vi "Autonomous Independent.vi"   [LabVIEW 2016]
doc: "This VI is called when autonomous begins, and will automatically be terminated when autonomous ends. You can carry out timed or sensor driven robot movement independently without needing to return to the caller."
uses:
  <vilib>/Rock Robotics/WPI/Solenoid/WPI_SolenoidValue.ctl
  <vilib>/Rock Robotics/WPI/Utilities/WPI_GetSetVariantRefNum.vi
  <vilib>/Rock Robotics/Network Tables/NT Read String.vi
  <vilib>/Rock Robotics/Network Tables/NT Write Numeric Array.vi
  <vilib>/Rock Robotics/Network Tables/NT Read Number.vi
  <vilib>/Rock Robotics/WPI/RobotDrive/WPI_RobotDriveArcadeDrive_Standard(NoSaturation).vi
  <vilib>/Rock Robotics/Network Tables/NT Write Number.vi
  <vilib>/Rock Robotics/Network Tables/NT Write String.vi
  <vilib>/Rock Robotics/WPI/Solenoid/WPI_SolenoidSetEnum.vi
  test2/Robot Global Data.vi
panel:
  # "Be sure to right-click and choose Data Operations>>Make Current Value default if you want to save the array values with the VI"
types:
  T1 = typedef "WPI_JoystickDevRef.ctl" = cluster{"Device":T2}
  T2 = typedef "WPI_JoystickDeviceEnum.ctl" = enum16{"USB 0", "USB 1", "USB 2", "USB 3", "USB 4", "USB 5"}
  T3 = typedef "WPI_EncoderDevRef.ctl" = cluster{"DevStatus":errorcluster, "EncoderIndex":T4, "CounterIndex":T5, "DistancePerCount":dbl, "Decoding Type":T6}
  T4 = typedef "FPGA_EncoderIdx.ctl" = enum8{"Enc 0", "Enc 1", "Enc 2", "Enc 3", "Enc 4", "Enc 5", "Enc 6", "Enc 7", "Invalid"}
  T5 = typedef "FPGA_CounterCtrSystemIndex.ctl" = enum8{"Ctr 0", "Ctr 1", "Ctr 2", "Ctr 3", "Ctr 4", "Ctr 5", "Ctr 6", "Ctr 7", "Invalid"}
  T6 = typedef "WPI_EncoderType.ctl" = enum16{"1x", "2x", "4x"}
  T7 = typedef "WPI_RobotDriveDevRef.ctl" = cluster{"DevStatus":errorcluster, "Motors[]":T8[], "Square Inputs":bool, "Max Output":dbl}
  T8 = typedef "WPI_MotorControlDeviceRef.ctl" = cluster{"DeviceStatus":errorcluster, "Type":T9, "PWM":cluster{"PWM Channel":T10, "DeadBand":T11}, "CAN":cluster{"Device Number":u8, "SetOutput VI Ref":variant, "GetOutput VI Ref":variant, "Enable VI Ref":variant, "Disable VI Ref":variant, "Data":variant}, "Invert":bool}
  T9 = typedef "WPI_MotorControlType.ctl" = enum16{"PWM", "CAN"}
  T10 = typedef "FPGA_DIOPWMChannel.ctl" = enum8{"PWM 0", "PWM 1", "PWM 2", "PWM 3", "PWM 4", "PWM 5", "PWM 6", "PWM 7", "PWM 8", "PWM 9", "PWM MXP 0", "PWM MXP 1", "PWM MXP 2", "PWM MXP 3", "PWM MXP 4", "PWM MXP 5", "PWM MXP 6", "PWM MXP 7", "PWM MXP 8", "PWM MXP 9", "Invalid"}
  T11 = typedef "WPI_PWMDeadband.ctl" = cluster{"Name":string, "maxPositivePwm":i32, "minPositivePwm":i32, "centerPwm":i32, "maxNegativePwm":i32, "minNegativePwm":i32, "angularRange":u16}
  T12 = typedef "WPI_GyroDevRef.ctl" = cluster{"DevStatus":errorcluster, "Analog Channel":T13, "Offset":dbl, "Gain (VoltsPerDegree/Second)":dbl, "Gyro Type":enum16{"Analog", "XRS450"}, "Handle":i32, "SPI Bus":T14, "Device Found":bool, "Sample Rate":dbl, "Calibrate On Open":bool}
  T13 = typedef "FPGA_AIChannel.ctl" = enum8{"AI 0", "AI 1", "AI 2", "AI 3", "AI MXP 0", "AI MXP 1", "AI MXP 2", "AI MXP 3", "Invalid"}
  T14 = typedef "spi_bus.ctl" = enum16{"SPI On-Board, CS0", "SPI On-Board, CS1", "SPI On-Board, CS2", "SPI On-Board, CS3", "SPI MXP", "Invalid"}
  T15 = typedef "WPI_SolenoidValue.ctl" = enum16{"Off", "On", "Forward", "Reverse"}
  T16 = typedef "WPI_SolenoidDevRef.ctl" = cluster{"DevStatus":errorcluster, "Pneumatics Control Module":u8, "Forward Solenoid Channel":T17, "Reverse Solenoid Channel":T17}
  T17 = typedef "WPI_SolenoidChannel.ctl" = enum8{"Solenoid 0", "Solenoid 1", "Solenoid 2", "Solenoid 3", "Solenoid 4", "Solenoid 5", "Solenoid 6", "Solenoid 7", "Invalid"}
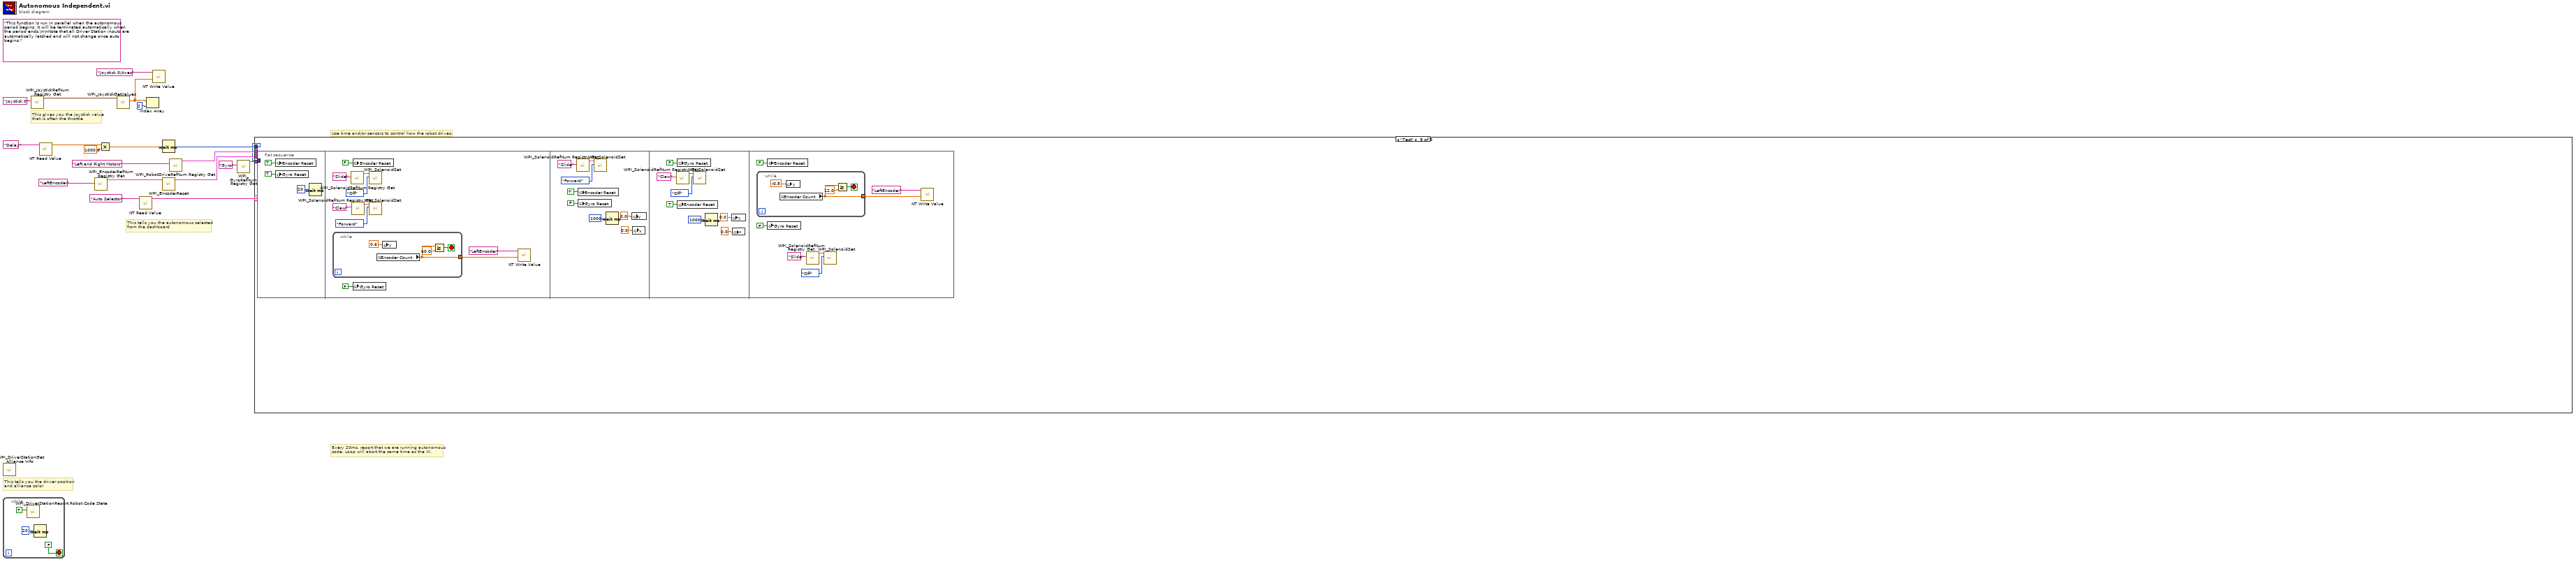
[diagram p0: block diagram]
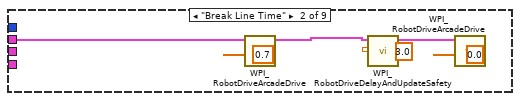
[diagram p3: hidden frame]
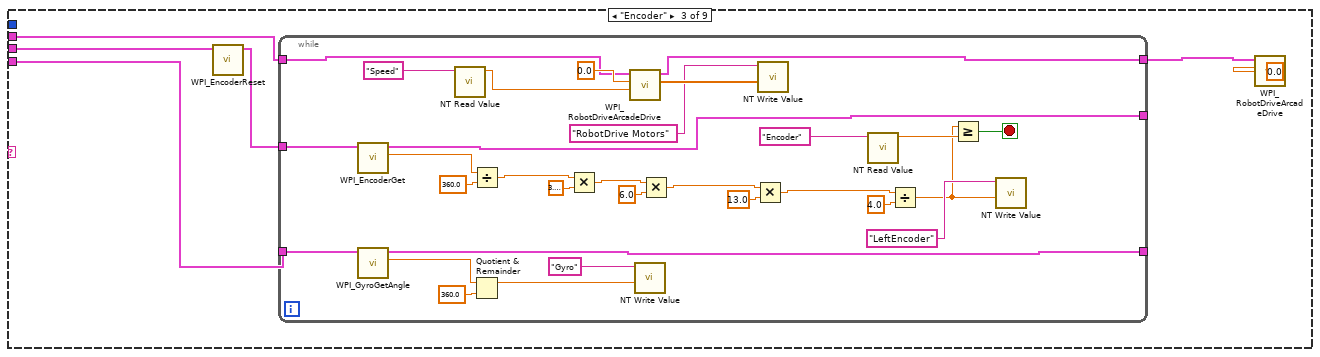
[diagram p4: hidden frame]
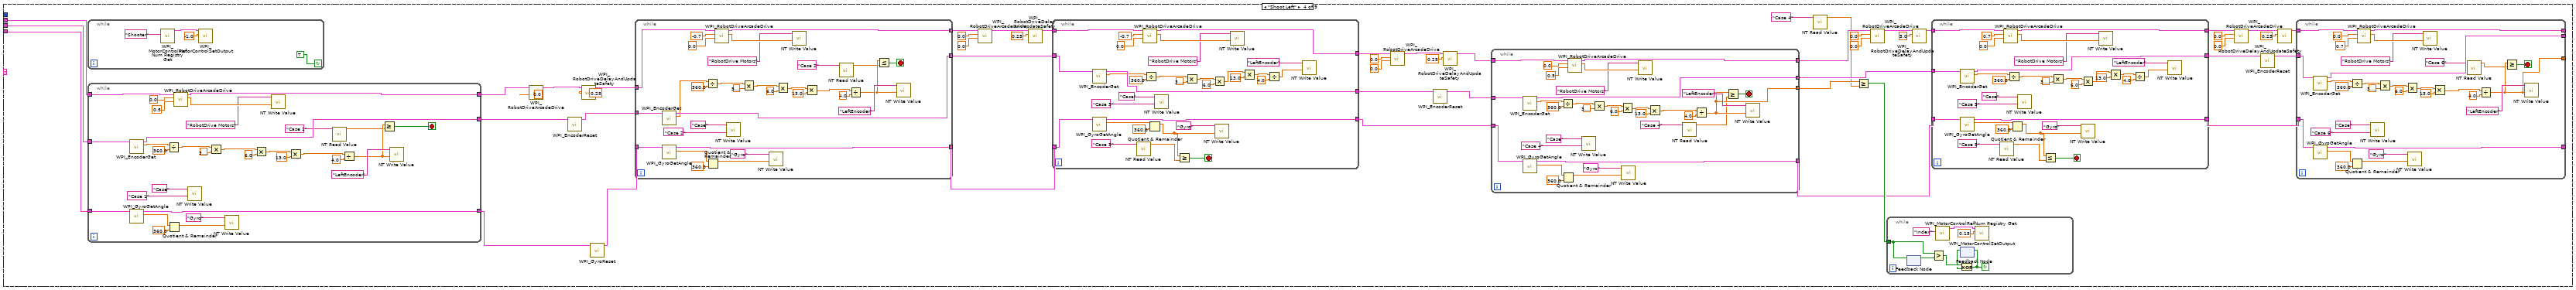
[diagram p5: hidden frame]
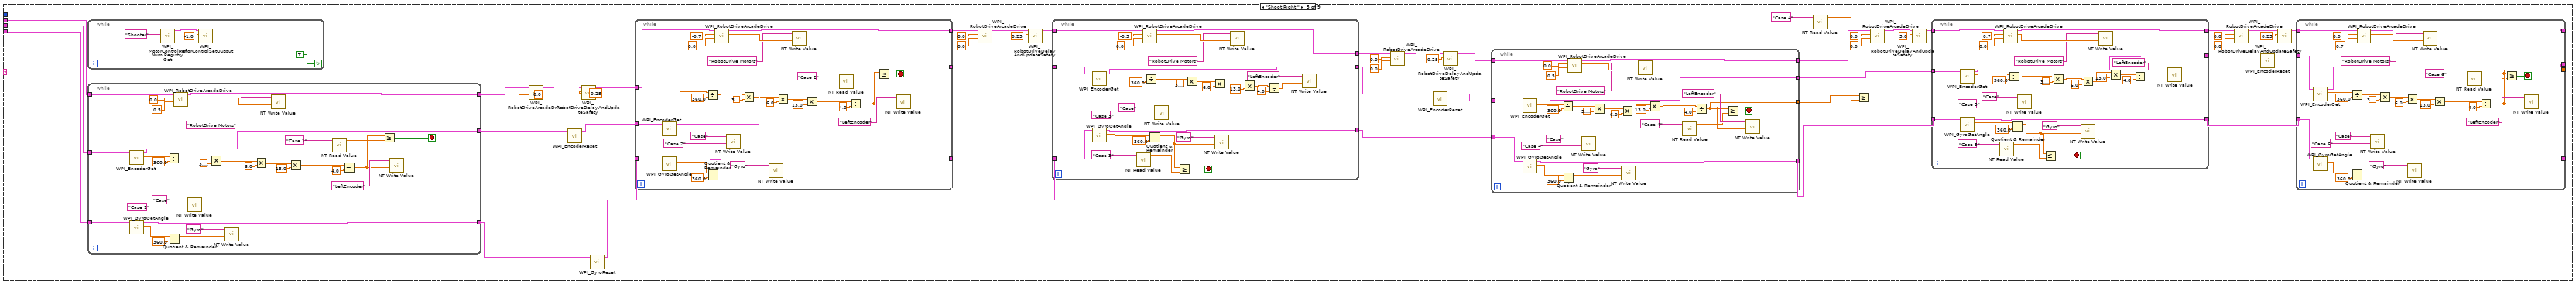
[diagram p6: hidden frame]
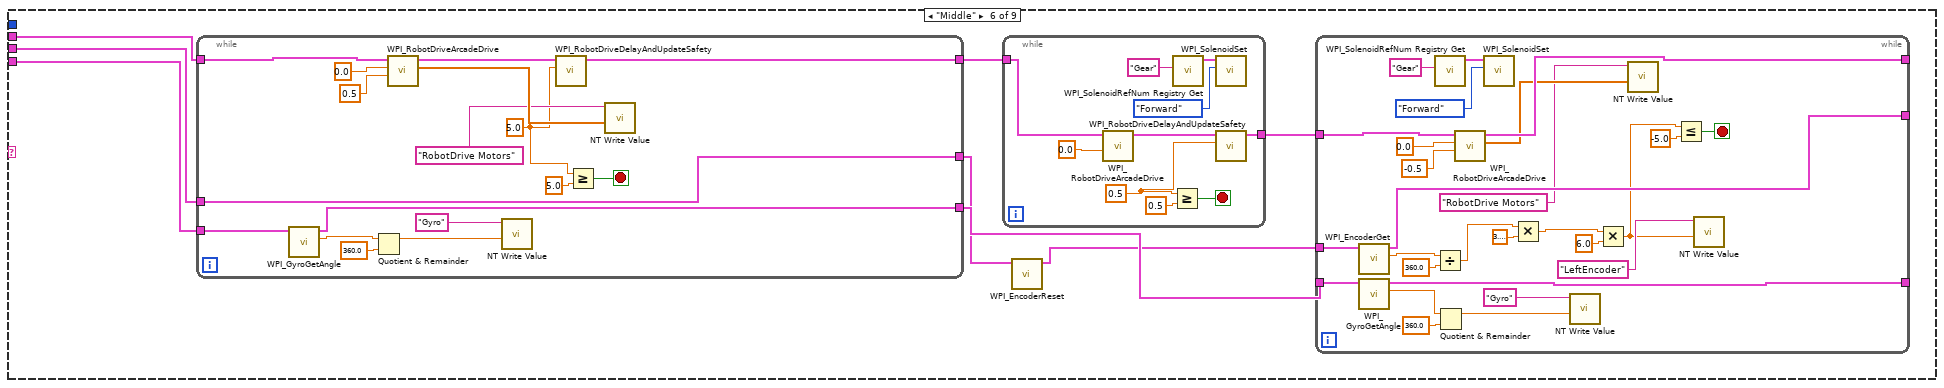
[diagram p7: hidden frame]
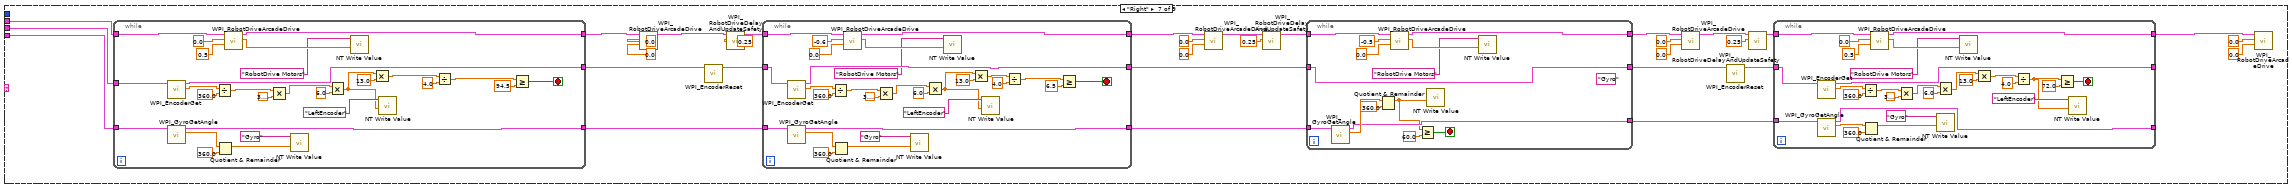
[diagram p8: hidden frame]
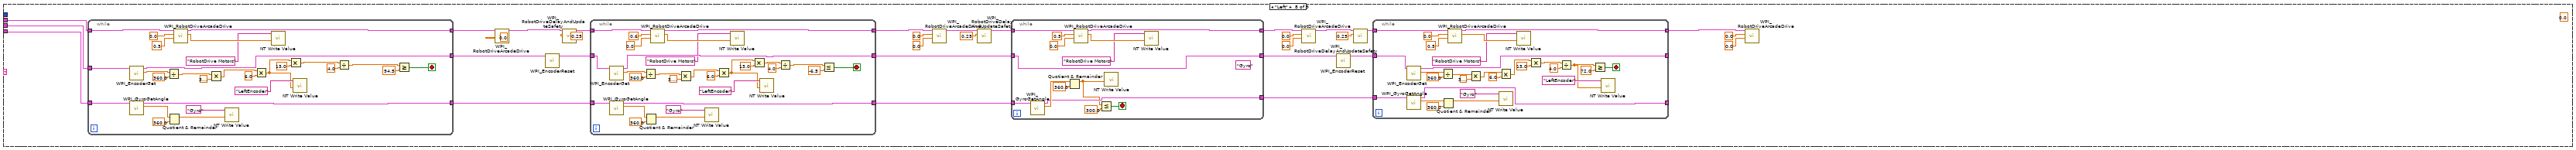
[diagram p9: hidden frame]
diagram:
  (unwired) "This function is run in parallel when the autonomous period begins. It will be terminated automatically when the period ends.\n\nNote that all Driver Station inputs are automatically latched and will not change once auto begins."
  # "This tells you the autonomous selected\nfrom the dashboard"
  # "Every 20ms, report that we are running autonomous\ncode. Loop will abort the same time as the VI."
  # "This gives you the joystick value\nthat is often the throttle"
  # "Use time and/or sensors to control how the robot drives."
  # "This tells you the driver position\nand alliance color"
  n1 = call <vilib>:"WPI_DriverStationGet Alliance Info.vi"() -> ()  [unwired: 12 out]
  n2 = while {
    stop <- FALSE stop-if-true
    n3 = call <vilib>:"WPI_DriverStationReport Robot Code State.vi"("Autonomous"=TRUE) -> ()  [unwired: 10 in, 1 out]
    n4 = Wait (ms)(milliseconds to wait=u32 20) -> ()  [unwired: 1 out]
  }
  n5 = call <vilib>:"WPI_JoystickRefNum Registry Get.vi"("refnum name"="Joystick 0") -> ("JoystickDevRef"=w18:T1)  [unwired: 1 in, 9 out]
  n6 = call-poly <vilib>:"NT Read Value.vi"("Name"="Delay") -> ("Numeric"=w7:dbl)  [unwired: 9 in, 1 out]
  n7 = call <vilib>:"WPI_EncoderRefNum Registry Get.vi"("refnum name"="LeftEncoder") -> ("EncoderDevRef"=w9:T3)  [unwired: 9 in, 1 out]
  n8 = Multiply(x=w7, y=1000.0) -> (x*y=w5:dbl)
  n9 = call <vilib>:"WPI_JoystickGetValues.vi"("JoystickDevRef"=w18) -> ("Axes"=w14:dbl[])  [unwired: 6 in, 4 out]
  n10 = call-poly <vilib>:"NT Read Value.vi"("Name"="Auto Selector") -> ("String"=w15:string)  [unwired: 9 in, 1 out]
  n11 = Index Array(array=w14, index=2) -> ()  [unwired: 1 out]
  n12 = call-poly <vilib>:"NT Write Value.vi"("Numeric Array"=w14, "Name"="Joystick 0/Axes") -> ()  [unwired: 9 in, 1 out]
  n13 = Wait (ms)(milliseconds to wait=w5) -> (millisecond timer value=w8:u32)
  n14 = call <vilib>:"WPI_EncoderReset.vi"("EncoderDevRef"=w9) -> ("EncoderDevRef"=w1:T3)  [unwired: 9 in, 1 out]
  n15 = call <vilib>:"WPI_RobotDriveRefNum Registry Get.vi"("refnum name"="Left and Right Motors") -> ("RobotDriveDevRef"=w3:T7)  [unwired: 1 in, 9 out]
  n16 = call <vilib>:"WPI_GyroRefNum Registry Get.vi"("refnum name"="Gyro") -> ("GyroDevRef"=w2:T12)  [unwired: 9 in, 1 out]
  n17 = case shown="\"Test\"" w15 {
    tunnel: w8 -> [_ _ _ _ _ _ _ _ w873]
    tunnel: w3 -> [_ w23 w33 w109 w315 w555 w626 w746 _]
    tunnel: w2 -> [_ _ w34 w108 w314 w554 w625 w745 _]
    tunnel: w1 -> [_ _ w32 w107 w313 w553 w624 w744 _]
    frame Default {
      # "You can put your main auto here, or you can right-click on the case and make any\nother frame be the default case."
      # "This is the frame that will execute if no selection is made, or if it is not recognized"
    }
    frame "Break Line Time" {
      n18 = call-poly <vilib>:"WPI_RobotDriveArcadeDrive.vi"("Y axis value"=0.7, "RobotDriveDevRef"=w23) -> ("RobotDriveDevRef"=w27:T7)  [unwired: 7 in, 2 out]
      n19 = call <vilib>:"WPI_RobotDriveDelayAndUpdateSafety.vi"("Delay (s)"=3.0, "RobotDriveDevRef"=w27) -> ("RobotDriveDevRef 2"=w25:T7)  [unwired: 8 in, 1 out]
      n20 = call-poly <vilib>:"WPI_RobotDriveArcadeDrive.vi"("Y axis value"=0.0, "RobotDriveDevRef"=w25) -> ()  [unwired: 7 in, 3 out]
    }
    frame "Encoder" {
      n21 = call <vilib>:"WPI_EncoderReset.vi"("EncoderDevRef"=w32) -> ("EncoderDevRef"=w29:T3)  [unwired: 9 in, 1 out]
      n22 = while {
        tunnel: [w62] -> _
        tunnel: [w61] -> w31
        tunnel: w33 -> [w43]
        tunnel: w34 -> [w42]
        tunnel: w29 -> [w41]
        tunnel: [w40] -> _
        stop <- w44 stop-if-true
        n23 = call <vilib>:"WPI_EncoderGet.vi"("EncoderDevRef"=w41) -> ("Distance"=w52:dbl, "EncoderDevRef"=w40:T3)  [unwired: 5 in, 4 out]
        n24 = call <vilib>:"WPI_GyroGetAngle.vi"("GyroDevRef"=w42) -> ("Angle"=w64:dbl, "GyroDevRef"=w62:T12)  [unwired: 6 in, 3 out]
        n25 = call-poly <vilib>:"NT Read Value.vi"("Name"="Speed") -> ("Numeric"=w35:dbl)  [unwired: 9 in, 1 out]
        n26 = Divide(x=w52, y=360.0) -> (x/y=w50:dbl)
        n27 = Quotient & Remainder(x=w64, y=360.0) -> (x-y*floor(x/y)=w60:dbl)  [unwired: 1 out]
        n28 = Multiply(x=w50, y=3.141592653589793) -> (x*y=w54:dbl)
        n29 = call-poly <vilib>:"WPI_RobotDriveArcadeDrive.vi"("Y axis value"=w35, "X axis value"=0.0, "RobotDriveDevRef"=w43) -> ("Motor Values"=w58:dbl[], "RobotDriveDevRef"=w61:T7)  [unwired: 6 in, 1 out]
        n30 = call-poly <vilib>:"NT Write Value.vi"("Numeric"=w60, "Name"="Gyro") -> ()  [unwired: 9 in, 1 out]
        n31 = Multiply(x=w54, y=6.0) -> (x*y=w45:dbl)
        n32 = Multiply(x=w45, y=13.0) -> (x*y=w46:dbl)
        n33 = call-poly <vilib>:"NT Write Value.vi"("Numeric Array"=w58, "Name"="RobotDrive Motors") -> ()  [unwired: 9 in, 1 out]
        n34 = call-poly <vilib>:"NT Read Value.vi"("Name"="Encoder") -> ("Numeric"=w39:dbl)  [unwired: 9 in, 1 out]
        n35 = Divide(x=w46, y=4.0) -> (x/y=w37:dbl)
        n36 = Greater Or Equal?(x=w37, y=w39) -> (x >= y?=w44:bool)
        n37 = call-poly <vilib>:"NT Write Value.vi"("Numeric"=w37, "Name"="LeftEncoder") -> ()  [unwired: 9 in, 1 out]
      }
      n38 = call-poly <vilib>:"WPI_RobotDriveArcadeDrive.vi"("X axis value"=0.0, "RobotDriveDevRef"=w31) -> ()  [unwired: 7 in, 3 out]
    }
    frame "Shoot Left" {
      n39 = while {
        stop <- TRUE ("x") continue-if-true
        n40 = call <vilib>:"WPI_MotorControlRefNum Registry Get.vi"("refnum name"="Shooter") -> ("MotorControlDevRef"=w179:T8)  [unwired: 9 in, 1 out]
        n41 = call <vilib>:"WPI_MotorControlSetOutput.vi"("Output"=-1.0, "MotorControlDevRef"=w179) -> ()  [unwired: 7 in, 3 out]
      }
      n42 = while {
        tunnel: [w308] -> w114
        tunnel: [w307] -> w96
        tunnel: [w306] -> w112
        tunnel: w109 -> [w289]
        tunnel: w108 -> [w288]
        tunnel: w107 -> [w287]
        stop <- w309 stop-if-true
        n43 = call <vilib>:"WPI_EncoderGet.vi"("EncoderDevRef"=w287) -> ("Distance"=w297:dbl, "EncoderDevRef"=w308:T3)  [unwired: 5 in, 4 out]
        n44 = call <vilib>:"WPI_GyroGetAngle.vi"("GyroDevRef"=w288) -> ("Angle"=w311:dbl, "GyroDevRef"=w307:T12)  [unwired: 6 in, 3 out]
        n45 = Divide(x=w297, y=360.0) -> (x/y=w295:dbl)
        n46 = Quotient & Remainder(x=w311, y=360.0) -> (x-y*floor(x/y)=w305:dbl)  [unwired: 1 out]
        n47 = call-poly <vilib>:"WPI_RobotDriveArcadeDrive.vi"("Y axis value"=0.5, "X axis value"=0.0, "RobotDriveDevRef"=w289) -> ("Motor Values"=w303:dbl[], "RobotDriveDevRef"=w306:T7)  [unwired: 6 in, 1 out]
        n48 = call-poly <vilib>:"NT Write Value.vi"("String"="Case 1", "Name"="Case") -> ()  [unwired: 9 in, 1 out]
        n49 = Multiply(x=w295, y=3.141592653589793) -> (x*y=w299:dbl)
        n50 = call-poly <vilib>:"NT Write Value.vi"("Numeric"=w305, "Name"="Gyro") -> ()  [unwired: 9 in, 1 out]
        n51 = Multiply(x=w299, y=6.0) -> (x*y=w290:dbl)
        n52 = call-poly <vilib>:"NT Write Value.vi"("Numeric Array"=w303, "Name"="RobotDrive Motors") -> ()  [unwired: 9 in, 1 out]
        n53 = Multiply(x=w290, y=13.0) -> (x*y=w291:dbl)
        n54 = call-poly <vilib>:"NT Read Value.vi"("Name"="Case 1") -> ("Numeric"=w284:dbl)  [unwired: 9 in, 1 out]
        n55 = Divide(x=w291, y=4.0) -> (x/y=w286:dbl)
        n56 = Greater Or Equal?(x=w286, y=w284) -> (x >= y?=w309:bool)
        n57 = call-poly <vilib>:"NT Write Value.vi"("Numeric"=w286, "Name"="LeftEncoder") -> ()  [unwired: 9 in, 1 out]
      }
      n58 = call-poly <vilib>:"WPI_RobotDriveArcadeDrive.vi"("Y axis value"=0.0, "RobotDriveDevRef"=w112) -> ("RobotDriveDevRef"=w111:T7)  [unwired: 7 in, 2 out]
      n59 = call <vilib>:"WPI_EncoderReset.vi"("EncoderDevRef"=w114) -> ("EncoderDevRef"=w105:T3)  [unwired: 9 in, 1 out]
      n60 = call <vilib>:"WPI_RobotDriveDelayAndUpdateSafety.vi"("Delay (s)"=0.25, "RobotDriveDevRef"=w111) -> ("RobotDriveDevRef 2"=w106:T7)  [unwired: 8 in, 1 out]
      n61 = call <vilib>:"WPI_GyroReset.vi"("GyroDevRef"=w96) -> ("GyroDevRef"=w95:T12)  [unwired: 9 in, 1 out]
      n62 = while {
        tunnel: [w278] -> w97
        tunnel: [w277] -> w98
        tunnel: [w276] -> w101
        tunnel: w106 -> [w259]
        tunnel: w95 -> [w258]
        tunnel: w105 -> [w257]
        stop <- w255 stop-if-true
        n63 = call <vilib>:"WPI_EncoderGet.vi"("EncoderDevRef"=w257) -> ("Distance"=w267:dbl, "EncoderDevRef"=w278:T3)  [unwired: 5 in, 4 out]
        n64 = call <vilib>:"WPI_GyroGetAngle.vi"("GyroDevRef"=w258) -> ("Angle"=w280:dbl, "GyroDevRef"=w277:T12)  [unwired: 6 in, 3 out]
        n65 = Divide(x=w267, y=360.0) -> (x/y=w265:dbl)
        n66 = Quotient & Remainder(x=w280, y=360.0) -> (x-y*floor(x/y)=w275:dbl)  [unwired: 1 out]
        n67 = call-poly <vilib>:"WPI_RobotDriveArcadeDrive.vi"("Y axis value"=0.0, "X axis value"=-0.7, "RobotDriveDevRef"=w259) -> ("Motor Values"=w273:dbl[], "RobotDriveDevRef"=w276:T7)  [unwired: 6 in, 1 out]
        n68 = call-poly <vilib>:"NT Write Value.vi"("String"="Case 2", "Name"="Case") -> ()  [unwired: 9 in, 1 out]
        n69 = Multiply(x=w265, y=3.141592653589793) -> (x*y=w269:dbl)
        n70 = call-poly <vilib>:"NT Write Value.vi"("Numeric"=w275, "Name"="Gyro") -> ()  [unwired: 9 in, 1 out]
        n71 = Multiply(x=w269, y=6.0) -> (x*y=w260:dbl)
        n72 = call-poly <vilib>:"NT Write Value.vi"("Numeric Array"=w273, "Name"="RobotDrive Motors") -> ()  [unwired: 9 in, 1 out]
        n73 = Multiply(x=w260, y=13.0) -> (x*y=w261:dbl)
        n74 = call-poly <vilib>:"NT Read Value.vi"("Name"="Case 2") -> ("Numeric"=w253:dbl)  [unwired: 9 in, 1 out]
        n75 = Divide(x=w261, y=4.0) -> (x/y=w256:dbl)
        n76 = Less Or Equal?(x=w256, y=w253) -> (x <= y?=w255:bool)
        n77 = call-poly <vilib>:"NT Write Value.vi"("Numeric"=w256, "Name"="LeftEncoder") -> ()  [unwired: 9 in, 1 out]
      }
      n78 = call-poly <vilib>:"WPI_RobotDriveArcadeDrive.vi"("Y axis value"=0.0, "X axis value"=0.0, "RobotDriveDevRef"=w101) -> ("RobotDriveDevRef"=w103:T7)  [unwired: 6 in, 2 out]
      n79 = call <vilib>:"WPI_RobotDriveDelayAndUpdateSafety.vi"("Delay (s)"=0.25, "RobotDriveDevRef"=w103) -> ("RobotDriveDevRef 2"=w99:T7)  [unwired: 8 in, 1 out]
      n80 = while {
        tunnel: [w246] -> w87
        tunnel: [w245] -> w88
        tunnel: [w244] -> w89
        tunnel: w99 -> [w228]
        tunnel: w98 -> [w227]
        tunnel: w97 -> [w226]
        stop <- w247 stop-if-true
        n81 = call <vilib>:"WPI_EncoderGet.vi"("EncoderDevRef"=w226) -> ("Distance"=w236:dbl, "EncoderDevRef"=w246:T3)  [unwired: 5 in, 4 out]
        n82 = call <vilib>:"WPI_GyroGetAngle.vi"("GyroDevRef"=w227) -> ("Angle"=w249:dbl, "GyroDevRef"=w245:T12)  [unwired: 6 in, 3 out]
        n83 = call-poly <vilib>:"NT Read Value.vi"("Name"="Case 3") -> ("Numeric"=w222:dbl)  [unwired: 9 in, 1 out]
        n84 = call-poly <vilib>:"WPI_RobotDriveArcadeDrive.vi"("Y axis value"=0.0, "X axis value"=-0.7, "RobotDriveDevRef"=w228) -> ("Motor Values"=w242:dbl[], "RobotDriveDevRef"=w244:T7)  [unwired: 6 in, 1 out]
        n85 = Divide(x=w236, y=360.0) -> (x/y=w234:dbl)
        n86 = Quotient & Remainder(x=w249, y=360.0) -> (x-y*floor(x/y)=w224:dbl)  [unwired: 1 out]
        n87 = call-poly <vilib>:"NT Write Value.vi"("String"="Case 3", "Name"="Case") -> ()  [unwired: 9 in, 1 out]
        n88 = Greater Or Equal?(x=w224, y=w222) -> (x >= y?=w247:bool)
        n89 = Multiply(x=w234, y=3.141592653589793) -> (x*y=w238:dbl)
        n90 = Multiply(x=w238, y=6.0) -> (x*y=w229:dbl)
        n91 = call-poly <vilib>:"NT Write Value.vi"("Numeric"=w224, "Name"="Gyro") -> ()  [unwired: 9 in, 1 out]
        n92 = call-poly <vilib>:"NT Write Value.vi"("Numeric Array"=w242, "Name"="RobotDrive Motors") -> ()  [unwired: 9 in, 1 out]
        n93 = Multiply(x=w229, y=13.0) -> (x*y=w230:dbl)
        n94 = Divide(x=w230, y=4.0) -> (x/y=w225:dbl)
        n95 = call-poly <vilib>:"NT Write Value.vi"("Numeric"=w225, "Name"="LeftEncoder") -> ()  [unwired: 9 in, 1 out]
      }
      n96 = call-poly <vilib>:"WPI_RobotDriveArcadeDrive.vi"("Y axis value"=0.0, "X axis value"=0.0, "RobotDriveDevRef"=w89) -> ("RobotDriveDevRef"=w93:T7)  [unwired: 6 in, 2 out]
      n97 = call <vilib>:"WPI_EncoderReset.vi"("EncoderDevRef"=w87) -> ("EncoderDevRef"=w86:T3)  [unwired: 9 in, 1 out]
      n98 = call <vilib>:"WPI_RobotDriveDelayAndUpdateSafety.vi"("Delay (s)"=0.25, "RobotDriveDevRef"=w93) -> ("RobotDriveDevRef 2"=w90:T7)  [unwired: 8 in, 1 out]
      n99 = while {
        tunnel: [w216] -> w82
        tunnel: [w215] -> w83
        tunnel: [w214] -> w78
        tunnel: w90 -> [w197]
        tunnel: w88 -> [w196]
        tunnel: w86 -> [w195]
        tunnel: [w193] -> w85
        stop <- w194 stop-if-true
        n100 = call <vilib>:"WPI_EncoderGet.vi"("EncoderDevRef"=w195) -> ("Distance"=w205:dbl, "EncoderDevRef"=w216:T3)  [unwired: 5 in, 4 out]
        n101 = call <vilib>:"WPI_GyroGetAngle.vi"("GyroDevRef"=w196) -> ("Angle"=w218:dbl, "GyroDevRef"=w215:T12)  [unwired: 6 in, 3 out]
        n102 = Divide(x=w205, y=360.0) -> (x/y=w203:dbl)
        n103 = Quotient & Remainder(x=w218, y=360.0) -> (x-y*floor(x/y)=w213:dbl)  [unwired: 1 out]
        n104 = call-poly <vilib>:"WPI_RobotDriveArcadeDrive.vi"("Y axis value"=0.5, "X axis value"=0.0, "RobotDriveDevRef"=w197) -> ("Motor Values"=w211:dbl[], "RobotDriveDevRef"=w214:T7)  [unwired: 6 in, 1 out]
        n105 = call-poly <vilib>:"NT Write Value.vi"("String"="Case 4", "Name"="Case") -> ()  [unwired: 9 in, 1 out]
        n106 = Multiply(x=w203, y=3.141592653589793) -> (x*y=w207:dbl)
        n107 = Multiply(x=w207, y=6.0) -> (x*y=w198:dbl)
        n108 = call-poly <vilib>:"NT Write Value.vi"("Numeric"=w213, "Name"="Gyro") -> ()  [unwired: 9 in, 1 out]
        n109 = call-poly <vilib>:"NT Write Value.vi"("Numeric Array"=w211, "Name"="RobotDrive Motors") -> ()  [unwired: 9 in, 1 out]
        n110 = Multiply(x=w198, y=13.0) -> (x*y=w199:dbl)
        n111 = call-poly <vilib>:"NT Read Value.vi"("Name"="Case 4") -> ("Numeric"=w191:dbl)  [unwired: 9 in, 1 out]
        n112 = Divide(x=w199, y=4.0) -> (x/y=w193:dbl)
        n113 = Greater Or Equal?(x=w193, y=w191) -> (x >= y?=w194:bool)
        n114 = call-poly <vilib>:"NT Write Value.vi"("Numeric"=w193, "Name"="LeftEncoder") -> ()  [unwired: 9 in, 1 out]
      }
      n115 = call-poly <vilib>:"NT Read Value.vi"("Name"="Case 4") -> ("Numeric"=w65:dbl)  [unwired: 9 in, 1 out]
      n116 = Greater Or Equal?(x=w85, y=w65) -> (x >= y?=w84:bool)
      n117 = call-poly <vilib>:"WPI_RobotDriveArcadeDrive.vi"("Y axis value"=0.0, "X axis value"=0.0, "RobotDriveDevRef"=w78) -> ("RobotDriveDevRef"=w80:T7)  [unwired: 6 in, 2 out]
      n118 = while {
        tunnel: w84 -> [w183]
        stop <- w182 continue-if-true
        n119 = feedback #1() -> (w186:bool)  [unwired: 1 in]
        n120 = feedback-in #1(w183) -> ()
        n121 = Greater?(x=w183, y=w186) -> (0:w185:bool)
        n122 = call <vilib>:"WPI_MotorControlRefNum Registry Get.vi"("refnum name"="Index") -> ("MotorControlDevRef"=w188:T8)  [unwired: 9 in, 1 out]
        n123 = feedback #2() -> (w184:bool)  [unwired: 1 in]
        n124 = Exclusive Or(1:w184, 2:w185) -> (0:w182:bool)
        n125 = feedback-in #2(w182) -> ()
        n126 = call <vilib>:"WPI_MotorControlSetOutput.vi"("Output"=0.15, "MotorControlDevRef"=w188) -> ()  [unwired: 7 in, 3 out]
      }
      n127 = call <vilib>:"WPI_RobotDriveDelayAndUpdateSafety.vi"("Delay (s)"=5.0, "RobotDriveDevRef"=w80) -> ("RobotDriveDevRef 2"=w76:T7)  [unwired: 8 in, 1 out]
      n128 = while {
        tunnel: [w173] -> w67
        tunnel: [w172] -> w68
        tunnel: [w171] -> w69
        tunnel: w76 -> [w155]
        tunnel: w83 -> [w154]
        tunnel: w82 -> [w151]
        stop <- w150 stop-if-true
        n129 = call <vilib>:"WPI_EncoderGet.vi"("EncoderDevRef"=w151) -> ("Distance"=w163:dbl, "EncoderDevRef"=w173:T3)  [unwired: 5 in, 4 out]
        n130 = call <vilib>:"WPI_GyroGetAngle.vi"("GyroDevRef"=w154) -> ("Angle"=w175:dbl, "GyroDevRef"=w172:T12)  [unwired: 6 in, 3 out]
        n131 = call-poly <vilib>:"NT Read Value.vi"("Name"="Case 5") -> ("Numeric"=w148:dbl)  [unwired: 9 in, 1 out]
        n132 = call-poly <vilib>:"WPI_RobotDriveArcadeDrive.vi"("Y axis value"=0.0, "X axis value"=0.7, "RobotDriveDevRef"=w155) -> ("Motor Values"=w169:dbl[], "RobotDriveDevRef"=w171:T7)  [unwired: 6 in, 1 out]
        n133 = Divide(x=w163, y=360.0) -> (x/y=w161:dbl)
        n134 = Quotient & Remainder(x=w175, y=360.0) -> (x-y*floor(x/y)=w152:dbl)  [unwired: 1 out]
        n135 = call-poly <vilib>:"NT Write Value.vi"("String"="Case 5", "Name"="Case") -> ()  [unwired: 9 in, 1 out]
        n136 = Less Or Equal?(x=w152, y=w148) -> (x <= y?=w150:bool)
        n137 = Multiply(x=w161, y=3.141592653589793) -> (x*y=w165:dbl)
        n138 = call-poly <vilib>:"NT Write Value.vi"("Numeric"=w152, "Name"="Gyro") -> ()  [unwired: 9 in, 1 out]
        n139 = Multiply(x=w165, y=6.0) -> (x*y=w156:dbl)
        n140 = call-poly <vilib>:"NT Write Value.vi"("Numeric Array"=w169, "Name"="RobotDrive Motors") -> ()  [unwired: 9 in, 1 out]
        n141 = Multiply(x=w156, y=13.0) -> (x*y=w157:dbl)
        n142 = Divide(x=w157, y=4.0) -> (x/y=w153:dbl)
        n143 = call-poly <vilib>:"NT Write Value.vi"("Numeric"=w153, "Name"="LeftEncoder") -> ()  [unwired: 9 in, 1 out]
      }
      n144 = call-poly <vilib>:"WPI_RobotDriveArcadeDrive.vi"("Y axis value"=0.0, "X axis value"=0.0, "RobotDriveDevRef"=w69) -> ("RobotDriveDevRef"=w74:T7)  [unwired: 6 in, 2 out]
      n145 = call <vilib>:"WPI_EncoderReset.vi"("EncoderDevRef"=w67) -> ("EncoderDevRef"=w70:T3)  [unwired: 9 in, 1 out]
      n146 = call <vilib>:"WPI_RobotDriveDelayAndUpdateSafety.vi"("Delay (s)"=0.25, "RobotDriveDevRef"=w74) -> ("RobotDriveDevRef 2"=w71:T7)  [unwired: 8 in, 1 out]
      n147 = while {
        tunnel: [w142] -> _
        tunnel: [w141] -> _
        tunnel: [w140] -> _
        tunnel: w71 -> [w123]
        tunnel: w68 -> [w122]
        tunnel: w70 -> [w121]
        tunnel: [w119] -> _
        stop <- w120 stop-if-true
        n148 = call <vilib>:"WPI_EncoderGet.vi"("EncoderDevRef"=w121) -> ("Distance"=w131:dbl, "EncoderDevRef"=w142:T3)  [unwired: 5 in, 4 out]
        n149 = call <vilib>:"WPI_GyroGetAngle.vi"("GyroDevRef"=w122) -> ("Angle"=w144:dbl, "GyroDevRef"=w141:T12)  [unwired: 6 in, 3 out]
        n150 = Divide(x=w131, y=360.0) -> (x/y=w129:dbl)
        n151 = Quotient & Remainder(x=w144, y=360.0) -> (x-y*floor(x/y)=w139:dbl)  [unwired: 1 out]
        n152 = call-poly <vilib>:"WPI_RobotDriveArcadeDrive.vi"("Y axis value"=0.7, "X axis value"=0.0, "RobotDriveDevRef"=w123) -> ("Motor Values"=w137:dbl[], "RobotDriveDevRef"=w140:T7)  [unwired: 6 in, 1 out]
        n153 = call-poly <vilib>:"NT Write Value.vi"("String"="Case 6", "Name"="Case") -> ()  [unwired: 9 in, 1 out]
        n154 = Multiply(x=w129, y=3.141592653589793) -> (x*y=w133:dbl)
        n155 = Multiply(x=w133, y=6.0) -> (x*y=w124:dbl)
        n156 = call-poly <vilib>:"NT Write Value.vi"("Numeric"=w139, "Name"="Gyro") -> ()  [unwired: 9 in, 1 out]
        n157 = call-poly <vilib>:"NT Write Value.vi"("Numeric Array"=w137, "Name"="RobotDrive Motors") -> ()  [unwired: 9 in, 1 out]
        n158 = Multiply(x=w124, y=13.0) -> (x*y=w125:dbl)
        n159 = call-poly <vilib>:"NT Read Value.vi"("Name"="Case 6") -> ("Numeric"=w117:dbl)  [unwired: 9 in, 1 out]
        n160 = Divide(x=w125, y=4.0) -> (x/y=w119:dbl)
        n161 = Greater Or Equal?(x=w119, y=w117) -> (x >= y?=w120:bool)
        n162 = call-poly <vilib>:"NT Write Value.vi"("Numeric"=w119, "Name"="LeftEncoder") -> ()  [unwired: 9 in, 1 out]
      }
    }
    frame "Shoot Right " {
      n163 = while {
        stop <- TRUE ("x") continue-if-true
        n164 = call <vilib>:"WPI_MotorControlRefNum Registry Get.vi"("refnum name"="Shooter") -> ("MotorControlDevRef"=w364:T8)  [unwired: 9 in, 1 out]
        n165 = call <vilib>:"WPI_MotorControlSetOutput.vi"("Output"=-1.0, "MotorControlDevRef"=w364) -> ()  [unwired: 7 in, 3 out]
      }
      n166 = while {
        tunnel: [w547] -> w361
        tunnel: [w546] -> w346
        tunnel: [w545] -> w359
        tunnel: w315 -> [w528]
        tunnel: w314 -> [w527]
        tunnel: w313 -> [w526]
        stop <- w548 stop-if-true
        n167 = call <vilib>:"WPI_EncoderGet.vi"("EncoderDevRef"=w526) -> ("Distance"=w536:dbl, "EncoderDevRef"=w547:T3)  [unwired: 5 in, 4 out]
        n168 = call <vilib>:"WPI_GyroGetAngle.vi"("GyroDevRef"=w527) -> ("Angle"=w550:dbl, "GyroDevRef"=w546:T12)  [unwired: 6 in, 3 out]
        n169 = Divide(x=w536, y=360.0) -> (x/y=w534:dbl)
        n170 = Quotient & Remainder(x=w550, y=360.0) -> (x-y*floor(x/y)=w544:dbl)  [unwired: 1 out]
        n171 = call-poly <vilib>:"WPI_RobotDriveArcadeDrive.vi"("Y axis value"=0.5, "X axis value"=0.0, "RobotDriveDevRef"=w528) -> ("Motor Values"=w542:dbl[], "RobotDriveDevRef"=w545:T7)  [unwired: 6 in, 1 out]
        n172 = call-poly <vilib>:"NT Write Value.vi"("String"="Case 1", "Name"="Case") -> ()  [unwired: 9 in, 1 out]
        n173 = Multiply(x=w534, y=3.141592653589793) -> (x*y=w538:dbl)
        n174 = call-poly <vilib>:"NT Write Value.vi"("Numeric"=w544, "Name"="Gyro") -> ()  [unwired: 9 in, 1 out]
        n175 = Multiply(x=w538, y=6.0) -> (x*y=w529:dbl)
        n176 = call-poly <vilib>:"NT Write Value.vi"("Numeric Array"=w542, "Name"="RobotDrive Motors") -> ()  [unwired: 9 in, 1 out]
        n177 = Multiply(x=w529, y=13.0) -> (x*y=w530:dbl)
        n178 = call-poly <vilib>:"NT Read Value.vi"("Name"="Case 1") -> ("Numeric"=w523:dbl)  [unwired: 9 in, 1 out]
        n179 = Divide(x=w530, y=4.0) -> (x/y=w525:dbl)
        n180 = Greater Or Equal?(x=w525, y=w523) -> (x >= y?=w548:bool)
        n181 = call-poly <vilib>:"NT Write Value.vi"("Numeric"=w525, "Name"="LeftEncoder") -> ()  [unwired: 9 in, 1 out]
      }
      n182 = call-poly <vilib>:"WPI_RobotDriveArcadeDrive.vi"("Y axis value"=0.0, "RobotDriveDevRef"=w359) -> ("RobotDriveDevRef"=w358:T7)  [unwired: 7 in, 2 out]
      n183 = call <vilib>:"WPI_EncoderReset.vi"("EncoderDevRef"=w361) -> ("EncoderDevRef"=w355:T3)  [unwired: 9 in, 1 out]
      n184 = call <vilib>:"WPI_RobotDriveDelayAndUpdateSafety.vi"("Delay (s)"=0.25, "RobotDriveDevRef"=w358) -> ("RobotDriveDevRef 2"=w356:T7)  [unwired: 8 in, 1 out]
      n185 = call <vilib>:"WPI_GyroReset.vi"("GyroDevRef"=w346) -> ("GyroDevRef"=w345:T12)  [unwired: 9 in, 1 out]
      n186 = while {
        tunnel: [w517] -> w347
        tunnel: [w516] -> w348
        tunnel: [w515] -> w351
        tunnel: w356 -> [w498]
        tunnel: w345 -> [w497]
        tunnel: w355 -> [w496]
        stop <- w494 stop-if-true
        n187 = call <vilib>:"WPI_EncoderGet.vi"("EncoderDevRef"=w496) -> ("Distance"=w506:dbl, "EncoderDevRef"=w517:T3)  [unwired: 5 in, 4 out]
        n188 = call <vilib>:"WPI_GyroGetAngle.vi"("GyroDevRef"=w497) -> ("Angle"=w519:dbl, "GyroDevRef"=w516:T12)  [unwired: 6 in, 3 out]
        n189 = Divide(x=w506, y=360.0) -> (x/y=w504:dbl)
        n190 = Quotient & Remainder(x=w519, y=360.0) -> (x-y*floor(x/y)=w514:dbl)  [unwired: 1 out]
        n191 = call-poly <vilib>:"WPI_RobotDriveArcadeDrive.vi"("Y axis value"=0.0, "X axis value"=-0.7, "RobotDriveDevRef"=w498) -> ("Motor Values"=w512:dbl[], "RobotDriveDevRef"=w515:T7)  [unwired: 6 in, 1 out]
        n192 = call-poly <vilib>:"NT Write Value.vi"("String"="Case 2", "Name"="Case") -> ()  [unwired: 9 in, 1 out]
        n193 = Multiply(x=w504, y=3.141592653589793) -> (x*y=w508:dbl)
        n194 = call-poly <vilib>:"NT Write Value.vi"("Numeric"=w514, "Name"="Gyro") -> ()  [unwired: 9 in, 1 out]
        n195 = Multiply(x=w508, y=6.0) -> (x*y=w499:dbl)
        n196 = call-poly <vilib>:"NT Write Value.vi"("Numeric Array"=w512, "Name"="RobotDrive Motors") -> ()  [unwired: 9 in, 1 out]
        n197 = Multiply(x=w499, y=13.0) -> (x*y=w500:dbl)
        n198 = call-poly <vilib>:"NT Read Value.vi"("Name"="Case 2") -> ("Numeric"=w492:dbl)  [unwired: 9 in, 1 out]
        n199 = Divide(x=w500, y=4.0) -> (x/y=w495:dbl)
        n200 = Less Or Equal?(x=w495, y=w492) -> (x <= y?=w494:bool)
        n201 = call-poly <vilib>:"NT Write Value.vi"("Numeric"=w495, "Name"="LeftEncoder") -> ()  [unwired: 9 in, 1 out]
      }
      n202 = call-poly <vilib>:"WPI_RobotDriveArcadeDrive.vi"("Y axis value"=0.0, "X axis value"=0.0, "RobotDriveDevRef"=w351) -> ("RobotDriveDevRef"=w353:T7)  [unwired: 6 in, 2 out]
      n203 = call <vilib>:"WPI_RobotDriveDelayAndUpdateSafety.vi"("Delay (s)"=0.25, "RobotDriveDevRef"=w353) -> ("RobotDriveDevRef 2"=w349:T7)  [unwired: 8 in, 1 out]
      n204 = while {
        tunnel: [w485] -> w337
        tunnel: [w484] -> w338
        tunnel: [w483] -> w339
        tunnel: w349 -> [w468]
        tunnel: w348 -> [w467]
        tunnel: w347 -> [w466]
        stop <- w486 stop-if-true
        n205 = call <vilib>:"WPI_EncoderGet.vi"("EncoderDevRef"=w466) -> ("Distance"=w459:dbl, "EncoderDevRef"=w485:T3)  [unwired: 5 in, 4 out]
        n206 = call <vilib>:"WPI_GyroGetAngle.vi"("GyroDevRef"=w467) -> ("Angle"=w488:dbl, "GyroDevRef"=w484:T12)  [unwired: 6 in, 3 out]
        n207 = call-poly <vilib>:"NT Read Value.vi"("Name"="Case 3") -> ("Numeric"=w462:dbl)  [unwired: 9 in, 1 out]
        n208 = call-poly <vilib>:"WPI_RobotDriveArcadeDrive.vi"("Y axis value"=0.0, "X axis value"=-0.5, "RobotDriveDevRef"=w468) -> ("Motor Values"=w481:dbl[], "RobotDriveDevRef"=w483:T7)  [unwired: 6 in, 1 out]
        n209 = Divide(x=w459, y=360.0) -> (x/y=w474:dbl)
        n210 = Quotient & Remainder(x=w488, y=360.0) -> (x-y*floor(x/y)=w464:dbl)  [unwired: 1 out]
        n211 = call-poly <vilib>:"NT Write Value.vi"("String"="Case 3", "Name"="Case") -> ()  [unwired: 9 in, 1 out]
        n212 = Greater Or Equal?(x=w464, y=w462) -> (x >= y?=w486:bool)
        n213 = Multiply(x=w474, y=3.141592653589793) -> (x*y=w477:dbl)
        n214 = Multiply(x=w477, y=6.0) -> (x*y=w469:dbl)
        n215 = call-poly <vilib>:"NT Write Value.vi"("Numeric"=w464, "Name"="Gyro") -> ()  [unwired: 9 in, 1 out]
        n216 = call-poly <vilib>:"NT Write Value.vi"("Numeric Array"=w481, "Name"="RobotDrive Motors") -> ()  [unwired: 9 in, 1 out]
        n217 = Multiply(x=w469, y=13.0) -> (x*y=w470:dbl)
        n218 = Divide(x=w470, y=4.0) -> (x/y=w465:dbl)
        n219 = call-poly <vilib>:"NT Write Value.vi"("Numeric"=w465, "Name"="LeftEncoder") -> ()  [unwired: 9 in, 1 out]
      }
      n220 = call-poly <vilib>:"WPI_RobotDriveArcadeDrive.vi"("Y axis value"=0.0, "X axis value"=0.0, "RobotDriveDevRef"=w339) -> ("RobotDriveDevRef"=w343:T7)  [unwired: 6 in, 2 out]
      n221 = call <vilib>:"WPI_EncoderReset.vi"("EncoderDevRef"=w337) -> ("EncoderDevRef"=w336:T3)  [unwired: 9 in, 1 out]
      n222 = call <vilib>:"WPI_RobotDriveDelayAndUpdateSafety.vi"("Delay (s)"=0.25, "RobotDriveDevRef"=w343) -> ("RobotDriveDevRef 2"=w340:T7)  [unwired: 8 in, 1 out]
      n223 = while {
        tunnel: [w455] -> w333
        tunnel: [w454] -> w334
        tunnel: [w453] -> w329
        tunnel: w340 -> [w436]
        tunnel: w338 -> [w435]
        tunnel: w336 -> [w434]
        tunnel: [w432] -> w335
        stop <- w433 stop-if-true
        n224 = call <vilib>:"WPI_EncoderGet.vi"("EncoderDevRef"=w434) -> ("Distance"=w444:dbl, "EncoderDevRef"=w455:T3)  [unwired: 5 in, 4 out]
        n225 = call <vilib>:"WPI_GyroGetAngle.vi"("GyroDevRef"=w435) -> ("Angle"=w457:dbl, "GyroDevRef"=w454:T12)  [unwired: 6 in, 3 out]
        n226 = Divide(x=w444, y=360.0) -> (x/y=w442:dbl)
        n227 = Quotient & Remainder(x=w457, y=360.0) -> (x-y*floor(x/y)=w452:dbl)  [unwired: 1 out]
        n228 = call-poly <vilib>:"WPI_RobotDriveArcadeDrive.vi"("Y axis value"=0.5, "X axis value"=0.0, "RobotDriveDevRef"=w436) -> ("Motor Values"=w450:dbl[], "RobotDriveDevRef"=w453:T7)  [unwired: 6 in, 1 out]
        n229 = call-poly <vilib>:"NT Write Value.vi"("String"="Case 4", "Name"="Case") -> ()  [unwired: 9 in, 1 out]
        n230 = Multiply(x=w442, y=3.141592653589793) -> (x*y=w446:dbl)
        n231 = Multiply(x=w446, y=6.0) -> (x*y=w437:dbl)
        n232 = call-poly <vilib>:"NT Write Value.vi"("Numeric"=w452, "Name"="Gyro") -> ()  [unwired: 9 in, 1 out]
        n233 = call-poly <vilib>:"NT Write Value.vi"("Numeric Array"=w450, "Name"="RobotDrive Motors") -> ()  [unwired: 9 in, 1 out]
        n234 = Multiply(x=w437, y=13.0) -> (x*y=w438:dbl)
        n235 = call-poly <vilib>:"NT Read Value.vi"("Name"="Case 4") -> ("Numeric"=w430:dbl)  [unwired: 9 in, 1 out]
        n236 = Divide(x=w438, y=4.0) -> (x/y=w432:dbl)
        n237 = Greater Or Equal?(x=w432, y=w430) -> (x >= y?=w433:bool)
        n238 = call-poly <vilib>:"NT Write Value.vi"("Numeric"=w432, "Name"="LeftEncoder") -> ()  [unwired: 9 in, 1 out]
      }
      n239 = call-poly <vilib>:"NT Read Value.vi"("Name"="Case 4") -> ("Numeric"=w316:dbl)  [unwired: 9 in, 1 out]
      n240 = Greater Or Equal?(x=w335, y=w316) -> ()  [unwired: 1 out]
      n241 = call-poly <vilib>:"WPI_RobotDriveArcadeDrive.vi"("Y axis value"=0.0, "X axis value"=0.0, "RobotDriveDevRef"=w329) -> ("RobotDriveDevRef"=w331:T7)  [unwired: 6 in, 2 out]
      n242 = call <vilib>:"WPI_RobotDriveDelayAndUpdateSafety.vi"("Delay (s)"=5.0, "RobotDriveDevRef"=w331) -> ("RobotDriveDevRef 2"=w327:T7)  [unwired: 8 in, 1 out]
      n243 = while {
        tunnel: [w424] -> w318
        tunnel: [w423] -> w319
        tunnel: [w422] -> w320
        tunnel: w327 -> [w406]
        tunnel: w334 -> [w405]
        tunnel: w333 -> [w402]
        stop <- w401 stop-if-true
        n244 = call <vilib>:"WPI_EncoderGet.vi"("EncoderDevRef"=w402) -> ("Distance"=w414:dbl, "EncoderDevRef"=w424:T3)  [unwired: 5 in, 4 out]
        n245 = call <vilib>:"WPI_GyroGetAngle.vi"("GyroDevRef"=w405) -> ("Angle"=w426:dbl, "GyroDevRef"=w423:T12)  [unwired: 6 in, 3 out]
        n246 = call-poly <vilib>:"NT Read Value.vi"("Name"="Case 5") -> ("Numeric"=w399:dbl)  [unwired: 9 in, 1 out]
        n247 = call-poly <vilib>:"WPI_RobotDriveArcadeDrive.vi"("Y axis value"=0.0, "X axis value"=0.7, "RobotDriveDevRef"=w406) -> ("Motor Values"=w420:dbl[], "RobotDriveDevRef"=w422:T7)  [unwired: 6 in, 1 out]
        n248 = Divide(x=w414, y=360.0) -> (x/y=w412:dbl)
        n249 = Quotient & Remainder(x=w426, y=360.0) -> (x-y*floor(x/y)=w403:dbl)  [unwired: 1 out]
        n250 = call-poly <vilib>:"NT Write Value.vi"("String"="Case 5", "Name"="Case") -> ()  [unwired: 9 in, 1 out]
        n251 = Less Or Equal?(x=w403, y=w399) -> (x <= y?=w401:bool)
        n252 = Multiply(x=w412, y=3.141592653589793) -> (x*y=w416:dbl)
        n253 = call-poly <vilib>:"NT Write Value.vi"("Numeric"=w403, "Name"="Gyro") -> ()  [unwired: 9 in, 1 out]
        n254 = Multiply(x=w416, y=6.0) -> (x*y=w407:dbl)
        n255 = call-poly <vilib>:"NT Write Value.vi"("Numeric Array"=w420, "Name"="RobotDrive Motors") -> ()  [unwired: 9 in, 1 out]
        n256 = Multiply(x=w407, y=13.0) -> (x*y=w408:dbl)
        n257 = Divide(x=w408, y=4.0) -> (x/y=w404:dbl)
        n258 = call-poly <vilib>:"NT Write Value.vi"("Numeric"=w404, "Name"="LeftEncoder") -> ()  [unwired: 9 in, 1 out]
      }
      n259 = call-poly <vilib>:"WPI_RobotDriveArcadeDrive.vi"("Y axis value"=0.0, "X axis value"=0.0, "RobotDriveDevRef"=w320) -> ("RobotDriveDevRef"=w325:T7)  [unwired: 6 in, 2 out]
      n260 = call <vilib>:"WPI_EncoderReset.vi"("EncoderDevRef"=w318) -> ("EncoderDevRef"=w321:T3)  [unwired: 9 in, 1 out]
      n261 = call <vilib>:"WPI_RobotDriveDelayAndUpdateSafety.vi"("Delay (s)"=0.25, "RobotDriveDevRef"=w325) -> ("RobotDriveDevRef 2"=w322:T7)  [unwired: 8 in, 1 out]
      n262 = while {
        tunnel: [w393] -> _
        tunnel: [w392] -> _
        tunnel: [w391] -> _
        tunnel: w322 -> [w374]
        tunnel: w319 -> [w373]
        tunnel: w321 -> [w372]
        tunnel: [w370] -> _
        stop <- w371 stop-if-true
        n263 = call <vilib>:"WPI_EncoderGet.vi"("EncoderDevRef"=w372) -> ("Distance"=w382:dbl, "EncoderDevRef"=w393:T3)  [unwired: 5 in, 4 out]
        n264 = call <vilib>:"WPI_GyroGetAngle.vi"("GyroDevRef"=w373) -> ("Angle"=w395:dbl, "GyroDevRef"=w392:T12)  [unwired: 6 in, 3 out]
        n265 = Divide(x=w382, y=360.0) -> (x/y=w380:dbl)
        n266 = Quotient & Remainder(x=w395, y=360.0) -> (x-y*floor(x/y)=w390:dbl)  [unwired: 1 out]
        n267 = call-poly <vilib>:"WPI_RobotDriveArcadeDrive.vi"("Y axis value"=0.7, "X axis value"=0.0, "RobotDriveDevRef"=w374) -> ("Motor Values"=w388:dbl[], "RobotDriveDevRef"=w391:T7)  [unwired: 6 in, 1 out]
        n268 = call-poly <vilib>:"NT Write Value.vi"("String"="Case 6", "Name"="Case") -> ()  [unwired: 9 in, 1 out]
        n269 = Multiply(x=w380, y=3.141592653589793) -> (x*y=w384:dbl)
        n270 = Multiply(x=w384, y=6.0) -> (x*y=w375:dbl)
        n271 = call-poly <vilib>:"NT Write Value.vi"("Numeric"=w390, "Name"="Gyro") -> ()  [unwired: 9 in, 1 out]
        n272 = call-poly <vilib>:"NT Write Value.vi"("Numeric Array"=w388, "Name"="RobotDrive Motors") -> ()  [unwired: 9 in, 1 out]
        n273 = Multiply(x=w375, y=13.0) -> (x*y=w376:dbl)
        n274 = call-poly <vilib>:"NT Read Value.vi"("Name"="Case 6") -> ("Numeric"=w368:dbl)  [unwired: 9 in, 1 out]
        n275 = Divide(x=w376, y=4.0) -> (x/y=w370:dbl)
        n276 = Greater Or Equal?(x=w370, y=w368) -> (x >= y?=w371:bool)
        n277 = call-poly <vilib>:"NT Write Value.vi"("Numeric"=w370, "Name"="LeftEncoder") -> ()  [unwired: 9 in, 1 out]
      }
    }
    frame "Middle" {
      n278 = while {
        tunnel: [w610] -> w559
        tunnel: [w603] -> w557
        tunnel: w555 -> [w599]
        tunnel: w554 -> [w598]
        tunnel: w553 -> [w597]
        tunnel: [w597] -> w552
        stop <- w602 stop-if-true
        w601 = 5.0 ("Delay (s)")
        n279 = call <vilib>:"WPI_GyroGetAngle.vi"("GyroDevRef"=w598) -> ("Angle"=w612:dbl, "GyroDevRef"=w610:T12)  [unwired: 6 in, 3 out]
        n280 = Quotient & Remainder(x=w612, y=360.0) -> (x-y*floor(x/y)=w609:dbl)  [unwired: 1 out]
        n281 = call-poly <vilib>:"WPI_RobotDriveArcadeDrive.vi"("Y axis value"=0.5, "X axis value"=0.0, "RobotDriveDevRef"=w599) -> ("Motor Values"=w607:dbl[], "RobotDriveDevRef"=w604:T7)  [unwired: 6 in, 1 out]
        n282 = call-poly <vilib>:"NT Write Value.vi"("Numeric"=w609, "Name"="Gyro") -> ()  [unwired: 9 in, 1 out]
        n283 = call <vilib>:"WPI_RobotDriveDelayAndUpdateSafety.vi"("Delay (s)"=w601, "RobotDriveDevRef"=w604) -> ("RobotDriveDevRef 2"=w603:T7)  [unwired: 8 in, 1 out]
        n284 = Greater Or Equal?(x=w601, y=5.0) -> (x >= y?=w602:bool)
        n285 = call-poly <vilib>:"NT Write Value.vi"("Numeric Array"=w607, "Name"="RobotDrive Motors") -> ()  [unwired: 9 in, 1 out]
      }
      n286 = while {
        tunnel: w557 -> [w567]
        tunnel: [w566] -> w556
        stop <- w563 stop-if-true
        w565 = 0.5 ("Delay (s)")
        n287 = call-poly <vilib>:"WPI_RobotDriveArcadeDrive.vi"("Y axis value"=0.0, "RobotDriveDevRef"=w567) -> ("RobotDriveDevRef"=w568:T7)  [unwired: 7 in, 2 out]
        n288 = Greater Or Equal?(x=w565, y=0.5) -> (x >= y?=w563:bool)
        n289 = call <vilib>:"WPI_SolenoidRefNum Registry Get.vi"("refnum name"="Gear") -> ("SolenoidDevRef"=w561:T16)  [unwired: 9 in, 1 out]
        n290 = call-poly <vilib>:"WPI_SolenoidSet.vi"("Value"=WPI_SolenoidValue."Forward", "SolenoidDevRef"=w561) -> ()  [unwired: 1 in, 9 out]
        n291 = call <vilib>:"WPI_RobotDriveDelayAndUpdateSafety.vi"("Delay (s)"=w565, "RobotDriveDevRef"=w568) -> ("RobotDriveDevRef 2"=w566:T7)  [unwired: 8 in, 1 out]
      }
      n292 = call <vilib>:"WPI_EncoderReset.vi"("EncoderDevRef"=w552) -> ("EncoderDevRef"=w558:T3)  [unwired: 9 in, 1 out]
      n293 = while {
        tunnel: w559 -> [w593]
        tunnel: [w592] -> _
        tunnel: [w591] -> _
        tunnel: [w590] -> _
        tunnel: w558 -> [w574]
        tunnel: w556 -> [w573]
        stop <- w575 stop-if-true
        n294 = call <vilib>:"WPI_EncoderGet.vi"("EncoderDevRef"=w574) -> ("Distance"=w580:dbl, "EncoderDevRef"=w592:T3)  [unwired: 5 in, 4 out]
        n295 = call <vilib>:"WPI_GyroGetAngle.vi"("GyroDevRef"=w593) -> ("Angle"=w595:dbl, "GyroDevRef"=w591:T12)  [unwired: 6 in, 3 out]
        n296 = call <vilib>:"WPI_SolenoidRefNum Registry Get.vi"("refnum name"="Gear") -> ("SolenoidDevRef"=w571:T16)  [unwired: 9 in, 1 out]
        n297 = Divide(x=w580, y=360.0) -> (x/y=w578:dbl)
        n298 = Quotient & Remainder(x=w595, y=360.0) -> (x-y*floor(x/y)=w588:dbl)  [unwired: 1 out]
        n299 = call-poly <vilib>:"WPI_RobotDriveArcadeDrive.vi"("Y axis value"=-0.5, "X axis value"=0.0, "RobotDriveDevRef"=w573) -> ("Motor Values"=w586:dbl[], "RobotDriveDevRef"=w590:T7)  [unwired: 6 in, 1 out]
        n300 = call-poly <vilib>:"WPI_SolenoidSet.vi"("Value"=WPI_SolenoidValue."Forward", "SolenoidDevRef"=w571) -> ()  [unwired: 1 in, 9 out]
        n301 = Multiply(x=w578, y=3.141592653589793) -> (x*y=w582:dbl)
        n302 = call-poly <vilib>:"NT Write Value.vi"("Numeric"=w588, "Name"="Gyro") -> ()  [unwired: 9 in, 1 out]
        n303 = Multiply(x=w582, y=6.0) -> (x*y=w576:dbl)
        n304 = call-poly <vilib>:"NT Write Value.vi"("Numeric Array"=w586, "Name"="RobotDrive Motors") -> ()  [unwired: 9 in, 1 out]
        n305 = Less Or Equal?(x=w576, y=-5.0) -> (x <= y?=w575:bool)
        n306 = call-poly <vilib>:"NT Write Value.vi"("Numeric"=w576, "Name"="LeftEncoder") -> ()  [unwired: 9 in, 1 out]
      }
    }
    frame "Right" {
      n307 = while {
        tunnel: [w739] -> w645
        tunnel: [w738] -> w643
        tunnel: [w737] -> w633
        tunnel: w626 -> [w718]
        tunnel: w625 -> [w717]
        tunnel: w624 -> [w716]
        stop <- w740 stop-if-true
        n308 = call <vilib>:"WPI_EncoderGet.vi"("EncoderDevRef"=w716) -> ("Distance"=w727:dbl, "EncoderDevRef"=w739:T3)  [unwired: 5 in, 4 out]
        n309 = call <vilib>:"WPI_GyroGetAngle.vi"("GyroDevRef"=w717) -> ("Angle"=w742:dbl, "GyroDevRef"=w738:T12)  [unwired: 6 in, 3 out]
        n310 = Divide(x=w727, y=360.0) -> (x/y=w725:dbl)
        n311 = Quotient & Remainder(x=w742, y=360.0) -> (x-y*floor(x/y)=w735:dbl)  [unwired: 1 out]
        n312 = call-poly <vilib>:"WPI_RobotDriveArcadeDrive.vi"("Y axis value"=0.5, "X axis value"=0.0, "RobotDriveDevRef"=w718) -> ("Motor Values"=w733:dbl[], "RobotDriveDevRef"=w737:T7)  [unwired: 6 in, 1 out]
        n313 = Multiply(x=w725, y=3.141592653589793) -> (x*y=w729:dbl)
        n314 = call-poly <vilib>:"NT Write Value.vi"("Numeric"=w735, "Name"="Gyro") -> ()  [unwired: 9 in, 1 out]
        n315 = Multiply(x=w729, y=6.0) -> (x*y=w720:dbl)
        n316 = call-poly <vilib>:"NT Write Value.vi"("Numeric Array"=w733, "Name"="RobotDrive Motors") -> ()  [unwired: 9 in, 1 out]
        n317 = Multiply(x=w720, y=13.0) -> (x*y=w721:dbl)
        n318 = call-poly <vilib>:"NT Write Value.vi"("Numeric"=w720, "Name"="LeftEncoder") -> ()  [unwired: 9 in, 1 out]
        n319 = Divide(x=w721, y=4.0) -> (x/y=w719:dbl)
        n320 = Greater Or Equal?(x=w719, y=94.5) -> (x >= y?=w740:bool)
      }
      n321 = call-poly <vilib>:"WPI_RobotDriveArcadeDrive.vi"("Y axis value"=0.0, "X axis value"=0.0, "RobotDriveDevRef"=w633) -> ("RobotDriveDevRef"=w632:T7)  [unwired: 6 in, 2 out]
      n322 = call <vilib>:"WPI_EncoderReset.vi"("EncoderDevRef"=w645) -> ("EncoderDevRef"=w644:T3)  [unwired: 9 in, 1 out]
      n323 = call <vilib>:"WPI_RobotDriveDelayAndUpdateSafety.vi"("Delay (s)"=0.25, "RobotDriveDevRef"=w632) -> ("RobotDriveDevRef 2"=w638:T7)  [unwired: 8 in, 1 out]
      n324 = while {
        tunnel: w638 -> [w685]
        tunnel: w643 -> [w698]
        tunnel: w644 -> [w697]
        tunnel: [w695] -> w642
        tunnel: [w694] -> w634
        tunnel: [w693] -> w630
        stop <- w696 stop-if-true
        n325 = call <vilib>:"WPI_EncoderGet.vi"("EncoderDevRef"=w697) -> ("Distance"=w682:dbl, "EncoderDevRef"=w695:T3)  [unwired: 5 in, 4 out]
        n326 = call <vilib>:"WPI_GyroGetAngle.vi"("GyroDevRef"=w698) -> ("Angle"=w700:dbl, "GyroDevRef"=w694:T12)  [unwired: 6 in, 3 out]
        n327 = Divide(x=w682, y=360.0) -> (x/y=w680:dbl)
        n328 = Quotient & Remainder(x=w700, y=360.0) -> (x-y*floor(x/y)=w691:dbl)  [unwired: 1 out]
        n329 = call-poly <vilib>:"WPI_RobotDriveArcadeDrive.vi"("Y axis value"=0.0, "X axis value"=-0.6, "RobotDriveDevRef"=w685) -> ("Motor Values"=w689:dbl[], "RobotDriveDevRef"=w693:T7)  [unwired: 6 in, 1 out]
        n330 = Multiply(x=w680, y=3.141592653589793) -> (x*y=w684:dbl)
        n331 = call-poly <vilib>:"NT Write Value.vi"("Numeric"=w691, "Name"="Gyro") -> ()  [unwired: 9 in, 1 out]
        n332 = Multiply(x=w684, y=6.0) -> (x*y=w676:dbl)
        n333 = call-poly <vilib>:"NT Write Value.vi"("Numeric Array"=w689, "Name"="RobotDrive Motors") -> ()  [unwired: 9 in, 1 out]
        n334 = Multiply(x=w676, y=13.0) -> (x*y=w677:dbl)
        n335 = call-poly <vilib>:"NT Write Value.vi"("Numeric"=w676, "Name"="LeftEncoder") -> ()  [unwired: 9 in, 1 out]
        n336 = Divide(x=w677, y=4.0) -> (x/y=w675:dbl)
        n337 = Greater Or Equal?(x=w675, y=6.5) -> (x >= y?=w696:bool)
      }
      n338 = call-poly <vilib>:"WPI_RobotDriveArcadeDrive.vi"("Y axis value"=0.0, "X axis value"=0.0, "RobotDriveDevRef"=w630) -> ("RobotDriveDevRef"=w629:T7)  [unwired: 6 in, 2 out]
      n339 = call <vilib>:"WPI_RobotDriveDelayAndUpdateSafety.vi"("Delay (s)"=0.25, "RobotDriveDevRef"=w629) -> ("RobotDriveDevRef 2"=w636:T7)  [unwired: 8 in, 1 out]
      n340 = while {
        tunnel: w634 -> [w713]
        tunnel: w642 -> [w702]
        tunnel: [w712] -> w641
        tunnel: w636 -> [w704]
        tunnel: [w703] -> w617
        tunnel: [w702] -> w640
        stop <- w709 stop-if-true
        (unwired) "Gyro" ("Name")
        n341 = call <vilib>:"WPI_GyroGetAngle.vi"("GyroDevRef"=w713) -> ("Angle"=w715:dbl, "GyroDevRef"=w712:T12)  [unwired: 6 in, 3 out]
        n342 = Quotient & Remainder(x=w715, y=360.0) -> (x-y*floor(x/y)=w711:dbl)  [unwired: 1 out]
        n343 = call-poly <vilib>:"WPI_RobotDriveArcadeDrive.vi"("Y axis value"=0.0, "X axis value"=-0.5, "RobotDriveDevRef"=w704) -> ("Motor Values"=w707:dbl[], "RobotDriveDevRef"=w703:T7)  [unwired: 6 in, 1 out]
        n344 = Greater Or Equal?(x=w711, y=60.0) -> (x >= y?=w709:bool)
        n345 = call-poly <vilib>:"NT Write Value.vi"("Numeric"=w711) -> ()  [unwired: 10 in, 1 out]
        n346 = call-poly <vilib>:"NT Write Value.vi"("Numeric Array"=w707, "Name"="RobotDrive Motors") -> ()  [unwired: 9 in, 1 out]
      }
      n347 = call-poly <vilib>:"WPI_RobotDriveArcadeDrive.vi"("Y axis value"=0.0, "X axis value"=0.0 ("Y axis value"), "RobotDriveDevRef"=w617) -> ("RobotDriveDevRef"=w620:T7)  [unwired: 6 in, 2 out]
      n348 = call <vilib>:"WPI_EncoderReset.vi"("EncoderDevRef"=w640) -> ("EncoderDevRef"=w639:T3)  [unwired: 9 in, 1 out]
      n349 = call <vilib>:"WPI_RobotDriveDelayAndUpdateSafety.vi"("Delay (s)"=0.25, "RobotDriveDevRef"=w620) -> ("RobotDriveDevRef 2"=w616:T7)  [unwired: 8 in, 1 out]
      n350 = while {
        tunnel: w616 -> [w658]
        tunnel: w641 -> [w670]
        tunnel: w639 -> [w669]
        tunnel: [w667] -> _
        tunnel: [w666] -> _
        tunnel: [w648] -> w628
        stop <- w668 stop-if-true
        n351 = call <vilib>:"WPI_EncoderGet.vi"("EncoderDevRef"=w669) -> ("Distance"=w655:dbl, "EncoderDevRef"=w667:T3)  [unwired: 5 in, 4 out]
        n352 = call <vilib>:"WPI_GyroGetAngle.vi"("GyroDevRef"=w670) -> ("Angle"=w672:dbl, "GyroDevRef"=w666:T12)  [unwired: 6 in, 3 out]
        n353 = Divide(x=w655, y=360.0) -> (x/y=w653:dbl)
        n354 = Quotient & Remainder(x=w672, y=360.0) -> (x-y*floor(x/y)=w664:dbl)  [unwired: 1 out]
        n355 = call-poly <vilib>:"WPI_RobotDriveArcadeDrive.vi"("Y axis value"=0.5, "X axis value"=0.0, "RobotDriveDevRef"=w658) -> ("Motor Values"=w662:dbl[], "RobotDriveDevRef"=w648:T7)  [unwired: 6 in, 1 out]
        n356 = Multiply(x=w653, y=3.141592653589793) -> (x*y=w657:dbl)
        n357 = call-poly <vilib>:"NT Write Value.vi"("Numeric"=w664, "Name"="Gyro") -> ()  [unwired: 9 in, 1 out]
        n358 = Multiply(x=w657, y=6.0) -> (x*y=w649:dbl)
        n359 = call-poly <vilib>:"NT Write Value.vi"("Numeric Array"=w662, "Name"="RobotDrive Motors") -> ()  [unwired: 9 in, 1 out]
        n360 = Multiply(x=w649, y=13.0) -> (x*y=w650:dbl)
        n361 = Divide(x=w650, y=4.0) -> (x/y=w646:dbl)
        n362 = Greater Or Equal?(x=w646, y=72.0) -> (x >= y?=w668:bool)
        n363 = call-poly <vilib>:"NT Write Value.vi"("Numeric"=w646, "Name"="LeftEncoder") -> ()  [unwired: 9 in, 1 out]
      }
      n364 = call-poly <vilib>:"WPI_RobotDriveArcadeDrive.vi"("Y axis value"=0.0, "X axis value"=0.0, "RobotDriveDevRef"=w628) -> ()  [unwired: 6 in, 3 out]
    }
    frame "Left" {
      (unwired) 0.0 ("X axis value")
      n365 = while {
        tunnel: [w868] -> w774
        tunnel: [w867] -> w772
        tunnel: [w866] -> w762
        tunnel: w746 -> [w847]
        tunnel: w745 -> [w846]
        tunnel: w744 -> [w845]
        stop <- w869 stop-if-true
        n366 = call <vilib>:"WPI_EncoderGet.vi"("EncoderDevRef"=w845) -> ("Distance"=w856:dbl, "EncoderDevRef"=w868:T3)  [unwired: 5 in, 4 out]
        n367 = call <vilib>:"WPI_GyroGetAngle.vi"("GyroDevRef"=w846) -> ("Angle"=w871:dbl, "GyroDevRef"=w867:T12)  [unwired: 6 in, 3 out]
        n368 = Divide(x=w856, y=360.0) -> (x/y=w854:dbl)
        n369 = Quotient & Remainder(x=w871, y=360.0) -> (x-y*floor(x/y)=w864:dbl)  [unwired: 1 out]
        n370 = call-poly <vilib>:"WPI_RobotDriveArcadeDrive.vi"("Y axis value"=0.5, "X axis value"=0.0, "RobotDriveDevRef"=w847) -> ("Motor Values"=w862:dbl[], "RobotDriveDevRef"=w866:T7)  [unwired: 6 in, 1 out]
        n371 = Multiply(x=w854, y=3.141592653589793) -> (x*y=w858:dbl)
        n372 = call-poly <vilib>:"NT Write Value.vi"("Numeric"=w864, "Name"="Gyro") -> ()  [unwired: 9 in, 1 out]
        n373 = Multiply(x=w858, y=6.0) -> (x*y=w849:dbl)
        n374 = call-poly <vilib>:"NT Write Value.vi"("Numeric Array"=w862, "Name"="RobotDrive Motors") -> ()  [unwired: 9 in, 1 out]
        n375 = Multiply(x=w849, y=13.0) -> (x*y=w850:dbl)
        n376 = call-poly <vilib>:"NT Write Value.vi"("Numeric"=w849, "Name"="LeftEncoder") -> ()  [unwired: 9 in, 1 out]
        n377 = Divide(x=w850, y=4.0) -> (x/y=w848:dbl)
        n378 = Greater Or Equal?(x=w848, y=94.5) -> (x >= y?=w869:bool)
      }
      n379 = call-poly <vilib>:"WPI_RobotDriveArcadeDrive.vi"("Y axis value"=0.0, "RobotDriveDevRef"=w762) -> ("RobotDriveDevRef"=w761:T7)  [unwired: 7 in, 2 out]
      n380 = call <vilib>:"WPI_EncoderReset.vi"("EncoderDevRef"=w774) -> ("EncoderDevRef"=w773:T3)  [unwired: 9 in, 1 out]
      n381 = call <vilib>:"WPI_RobotDriveDelayAndUpdateSafety.vi"("Delay (s)"=0.25, "RobotDriveDevRef"=w761) -> ("RobotDriveDevRef 2"=w767:T7)  [unwired: 8 in, 1 out]
      n382 = while {
        tunnel: w767 -> [w814]
        tunnel: w772 -> [w827]
        tunnel: w773 -> [w826]
        tunnel: [w824] -> w771
        tunnel: [w823] -> w763
        tunnel: [w822] -> w759
        stop <- w825 stop-if-true
        n383 = call <vilib>:"WPI_EncoderGet.vi"("EncoderDevRef"=w826) -> ("Distance"=w811:dbl, "EncoderDevRef"=w824:T3)  [unwired: 5 in, 4 out]
        n384 = call <vilib>:"WPI_GyroGetAngle.vi"("GyroDevRef"=w827) -> ("Angle"=w829:dbl, "GyroDevRef"=w823:T12)  [unwired: 6 in, 3 out]
        n385 = Divide(x=w811, y=360.0) -> (x/y=w809:dbl)
        n386 = Quotient & Remainder(x=w829, y=360.0) -> (x-y*floor(x/y)=w820:dbl)  [unwired: 1 out]
        n387 = call-poly <vilib>:"WPI_RobotDriveArcadeDrive.vi"("Y axis value"=0.0, "X axis value"=0.6, "RobotDriveDevRef"=w814) -> ("Motor Values"=w818:dbl[], "RobotDriveDevRef"=w822:T7)  [unwired: 6 in, 1 out]
        n388 = Multiply(x=w809, y=3.141592653589793) -> (x*y=w813:dbl)
        n389 = call-poly <vilib>:"NT Write Value.vi"("Numeric"=w820, "Name"="Gyro") -> ()  [unwired: 9 in, 1 out]
        n390 = Multiply(x=w813, y=6.0) -> (x*y=w805:dbl)
        n391 = call-poly <vilib>:"NT Write Value.vi"("Numeric Array"=w818, "Name"="RobotDrive Motors") -> ()  [unwired: 9 in, 1 out]
        n392 = Multiply(x=w805, y=13.0) -> (x*y=w806:dbl)
        n393 = call-poly <vilib>:"NT Write Value.vi"("Numeric"=w805, "Name"="LeftEncoder") -> ()  [unwired: 9 in, 1 out]
        n394 = Divide(x=w806, y=4.0) -> (x/y=w804:dbl)
        n395 = Less Or Equal?(x=w804, y=-6.5) -> (x <= y?=w825:bool)
      }
      n396 = call-poly <vilib>:"WPI_RobotDriveArcadeDrive.vi"("Y axis value"=0.0, "X axis value"=0.0, "RobotDriveDevRef"=w759) -> ("RobotDriveDevRef"=w758:T7)  [unwired: 6 in, 2 out]
      n397 = call <vilib>:"WPI_RobotDriveDelayAndUpdateSafety.vi"("Delay (s)"=0.25, "RobotDriveDevRef"=w758) -> ("RobotDriveDevRef 2"=w765:T7)  [unwired: 8 in, 1 out]
      n398 = while {
        tunnel: w763 -> [w842]
        tunnel: w771 -> [w831]
        tunnel: [w841] -> w770
        tunnel: w765 -> [w833]
        tunnel: [w832] -> w749
        tunnel: [w831] -> w769
        stop <- w838 stop-if-true
        (unwired) "Gyro" ("Name")
        n399 = call <vilib>:"WPI_GyroGetAngle.vi"("GyroDevRef"=w842) -> ("Angle"=w844:dbl, "GyroDevRef"=w841:T12)  [unwired: 6 in, 3 out]
        n400 = Quotient & Remainder(x=w844, y=360.0) -> (x-y*floor(x/y)=w840:dbl)  [unwired: 1 out]
        n401 = call-poly <vilib>:"WPI_RobotDriveArcadeDrive.vi"("Y axis value"=0.0, "X axis value"=0.5, "RobotDriveDevRef"=w833) -> ("Motor Values"=w836:dbl[], "RobotDriveDevRef"=w832:T7)  [unwired: 6 in, 1 out]
        n402 = Less Or Equal?(x=w840, y=300.0) -> (x <= y?=w838:bool)
        n403 = call-poly <vilib>:"NT Write Value.vi"("Numeric"=w840) -> ()  [unwired: 10 in, 1 out]
        n404 = call-poly <vilib>:"NT Write Value.vi"("Numeric Array"=w836, "Name"="RobotDrive Motors") -> ()  [unwired: 9 in, 1 out]
      }
      n405 = call-poly <vilib>:"WPI_RobotDriveArcadeDrive.vi"("Y axis value"=0.0, "X axis value"=0.0 ("Y axis value"), "RobotDriveDevRef"=w749) -> ("RobotDriveDevRef"=w752:T7)  [unwired: 6 in, 2 out]
      n406 = call <vilib>:"WPI_EncoderReset.vi"("EncoderDevRef"=w769) -> ("EncoderDevRef"=w768:T3)  [unwired: 9 in, 1 out]
      n407 = call <vilib>:"WPI_RobotDriveDelayAndUpdateSafety.vi"("Delay (s)"=0.25, "RobotDriveDevRef"=w752) -> ("RobotDriveDevRef 2"=w748:T7)  [unwired: 8 in, 1 out]
      n408 = while {
        tunnel: w748 -> [w787]
        tunnel: w770 -> [w799]
        tunnel: w768 -> [w798]
        tunnel: [w796] -> _
        tunnel: [w795] -> _
        tunnel: [w777] -> w757
        stop <- w797 stop-if-true
        n409 = call <vilib>:"WPI_EncoderGet.vi"("EncoderDevRef"=w798) -> ("Distance"=w784:dbl, "EncoderDevRef"=w796:T3)  [unwired: 5 in, 4 out]
        n410 = call <vilib>:"WPI_GyroGetAngle.vi"("GyroDevRef"=w799) -> ("Angle"=w801:dbl, "GyroDevRef"=w795:T12)  [unwired: 6 in, 3 out]
        n411 = Divide(x=w784, y=360.0) -> (x/y=w782:dbl)
        n412 = Quotient & Remainder(x=w801, y=360.0) -> (x-y*floor(x/y)=w793:dbl)  [unwired: 1 out]
        n413 = call-poly <vilib>:"WPI_RobotDriveArcadeDrive.vi"("Y axis value"=0.5, "X axis value"=0.0, "RobotDriveDevRef"=w787) -> ("Motor Values"=w791:dbl[], "RobotDriveDevRef"=w777:T7)  [unwired: 6 in, 1 out]
        n414 = Multiply(x=w782, y=3.141592653589793) -> (x*y=w786:dbl)
        n415 = call-poly <vilib>:"NT Write Value.vi"("Numeric"=w793, "Name"="Gyro") -> ()  [unwired: 9 in, 1 out]
        n416 = Multiply(x=w786, y=6.0) -> (x*y=w778:dbl)
        n417 = call-poly <vilib>:"NT Write Value.vi"("Numeric Array"=w791, "Name"="RobotDrive Motors") -> ()  [unwired: 9 in, 1 out]
        n418 = Multiply(x=w778, y=13.0) -> (x*y=w779:dbl)
        n419 = Divide(x=w779, y=4.0) -> (x/y=w775:dbl)
        n420 = Greater Or Equal?(x=w775, y=72.0) -> (x >= y?=w797:bool)
        n421 = call-poly <vilib>:"NT Write Value.vi"("Numeric"=w775, "Name"="LeftEncoder") -> ()  [unwired: 9 in, 1 out]
      }
      n422 = call-poly <vilib>:"WPI_RobotDriveArcadeDrive.vi"("Y axis value"=0.0, "X axis value"=0.0, "RobotDriveDevRef"=w757) -> ()  [unwired: 6 in, 3 out]
    }
    frame "Test" {
      n423 = flat-sequence {
        tunnel: w873 -> [_]
        frame #0 {
          n424 = global write "Robot Global Data.vi" "Encoder Reset"(TRUE ("Encoder Reset")) -> ()
          n425 = global write "Robot Global Data.vi" "Gyro Reset"(TRUE ("Gyro Reset")) -> ()
          n426 = Wait (ms)(milliseconds to wait=u32 20) -> ()  [unwired: 1 out]
        }
        frame #1 {
          n427 = while {
            tunnel: [w888] -> w883
            stop <- w890 stop-if-true
            n428 = global read "Robot Global Data.vi" "Encoder Count"() -> (w888:dbl)
            n429 = global write "Robot Global Data.vi" "y"(0.6 ("Drive Speed")) -> ()
            n430 = Greater Or Equal?(x=w888, y=60.0) -> (x >= y?=w890:bool)
          }
          n431 = call <vilib>:"WPI_SolenoidRefNum Registry Get.vi"("refnum name"="Slide") -> ("SolenoidDevRef"=w882:T16)  [unwired: 9 in, 1 out]
          n432 = call <vilib>:"WPI_SolenoidRefNum Registry Get.vi"("refnum name"="Claw") -> ("SolenoidDevRef"=w879:T16)  [unwired: 9 in, 1 out]
          n433 = global write "Robot Global Data.vi" "Encoder Reset"(FALSE ("Encoder Reset")) -> ()
          n434 = global write "Robot Global Data.vi" "Gyro Reset"(FALSE ("Gyro Reset")) -> ()
          n435 = call-poly <vilib>:"WPI_SolenoidSet.vi"("Value"=WPI_SolenoidValue."Off", "SolenoidDevRef"=w882) -> ()  [unwired: 1 in, 9 out]
          n436 = call-poly <vilib>:"WPI_SolenoidSet.vi"("Value"=WPI_SolenoidValue."Forward", "SolenoidDevRef"=w879) -> ()  [unwired: 1 in, 9 out]
          n437 = call-poly <vilib>:"NT Write Value.vi"("Numeric"=w883, "Name"="LeftEncoder") -> ()  [unwired: 9 in, 1 out]
        }
        frame #2 {
          n438 = call <vilib>:"WPI_SolenoidRefNum Registry Get.vi"("refnum name"="Slide") -> ("SolenoidDevRef"=w891:T16)  [unwired: 9 in, 1 out]
          n439 = global write "Robot Global Data.vi" "Encoder Reset"(TRUE ("Encoder Reset")) -> ()
          n440 = global write "Robot Global Data.vi" "Gyro Reset"(FALSE ("Gyro Reset")) -> ()
          n441 = call-poly <vilib>:"WPI_SolenoidSet.vi"("Value"=WPI_SolenoidValue."Forward", "SolenoidDevRef"=w891) -> ()  [unwired: 1 in, 9 out]
          n442 = Wait (ms)(milliseconds to wait=u32 1000) -> ()  [unwired: 1 out]
          n443 = global write "Robot Global Data.vi" "y"(0.0 ("Drive Speed")) -> ()
          n444 = global write "Robot Global Data.vi" "x"(0.0) -> ()
        }
        frame #3 {
          n445 = call <vilib>:"WPI_SolenoidRefNum Registry Get.vi"("refnum name"="Claw") -> ("SolenoidDevRef"=w905:T16)  [unwired: 9 in, 1 out]
          n446 = global write "Robot Global Data.vi" "Gyro Reset"(FALSE ("Gyro Reset")) -> ()
          n447 = global write "Robot Global Data.vi" "Encoder Reset"(TRUE ("Encoder Reset")) -> ()
          n448 = call-poly <vilib>:"WPI_SolenoidSet.vi"("Value"=WPI_SolenoidValue."Off", "SolenoidDevRef"=w905) -> ()  [unwired: 1 in, 9 out]
          n449 = Wait (ms)(milliseconds to wait=u32 1000) -> ()  [unwired: 1 out]
          n450 = global write "Robot Global Data.vi" "y"(0.0 ("Drive Speed")) -> ()
          n451 = global write "Robot Global Data.vi" "x"(0.0) -> ()
        }
        frame #4 {
          n452 = while {
            tunnel: [w915] -> w910
            stop <- w917 stop-if-true
            n453 = global read "Robot Global Data.vi" "Encoder Count"() -> (w915:dbl)
            n454 = global write "Robot Global Data.vi" "y"(-0.5 ("Drive Speed")) -> ()
            n455 = Greater Or Equal?(x=w915, y=12.0) -> (x >= y?=w917:bool)
          }
          n456 = global write "Robot Global Data.vi" "Encoder Reset"(FALSE ("Encoder Reset")) -> ()
          n457 = global write "Robot Global Data.vi" "Gyro Reset"(FALSE ("Gyro Reset")) -> ()
          n458 = call <vilib>:"WPI_SolenoidRefNum Registry Get.vi"("refnum name"="Slide") -> ("SolenoidDevRef"=w907:T16)  [unwired: 9 in, 1 out]
          n459 = call-poly <vilib>:"WPI_SolenoidSet.vi"("Value"=WPI_SolenoidValue."Off", "SolenoidDevRef"=w907) -> ()  [unwired: 1 in, 9 out]
          n460 = call-poly <vilib>:"NT Write Value.vi"("Numeric"=w910, "Name"="LeftEncoder") -> ()  [unwired: 9 in, 1 out]
        }
      }
    }
  }
